vi "Msg Specific.vi"   [LabVIEW 2020, in "jettl.lvlib" / "Msg Specific.lvlib"]
uses:
  Msg Specific.lvlib
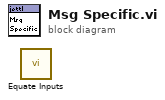
[diagram p0: block diagram]
diagram:
  n1 = call "Equate Inputs.vi"() -> ()  [unwired: 11 in, 1 out]
